vi "Get Add Package Command.vi"(8 "error in (no error)":errorcluster) -> (0 "error out":errorcluster, 3 "Add Package to Feed Command":string)   [LabVIEW 2014, in "NIPM_API.lvlib"]
doc: "Returns the NIPM version correct command to add package(s) to a feed"
uses:
  NIPM_API.lvlib
  Version Comparison Operator.ctl
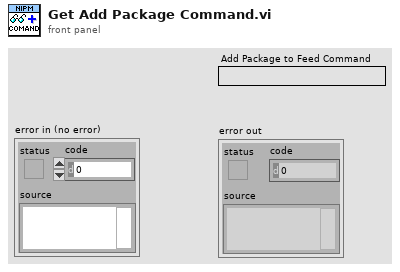
[diagram p1: front panel]
types:
  T1 = typedef "NIPM_API.lvlib/Version Comparison Operator.ctl" = enum16{">", ">=", "=", "!=", "<=", "<"}
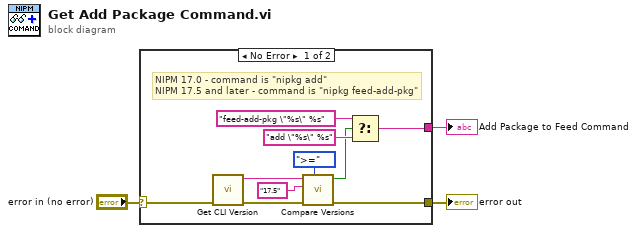
[diagram p0: block diagram]
diagram:
  n1 = case shown="No Error" "error in (no error)" {
    selector: "error in (no error)" -> [w9 w14]
    tunnel: [w8 w14] -> w3
    tunnel: [w4 _] -> w1
    frame No Error {
      # "NIPM 17.0 - command is \"nipkg add\"\nNIPM 17.5 and later - command is \"nipkg feed-add-pkg\""
      n2 = call "Get CLI Version.vi"("error in"=w9) -> ("error out"=w13:errorcluster, "full version string"=w10:string)  [unwired: 9 in]
      n3 = call "Compare Versions.vi"("operator"=Version_Comparison_Operator.">=", "error in"=w13, "version y"="17.5", "version x"=w10) -> ("error out"=w8:errorcluster, "Satisfied?"=w5:bool)  [unwired: 6 in]
      n4 = Select(t="feed-add-pkg \"%s\" %s" ("format string"), s=w5, f="add \"%s\" %s" ("format string")) -> (s? t:f=w4:string)
    }
    frame Error {
    }
  }
  "error out" <- w3
  "Add Package to Feed Command" <- w1
